vi "Joystick_Normalize.vi"(11 "Joystick In":i8) -> (3 "Norm Out":dbl)   [LabVIEW 2012]
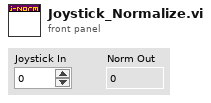
[diagram p1: front panel]
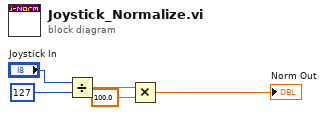
[diagram p0: block diagram]
diagram:
  n1 = Divide(x="Joystick In", y=i8 127) -> (x/y=w2:dbl)
  n2 = Multiply(x=w2, y=100.0) -> (x*y=→"Norm Out":dbl)
